vi "Global INIT.vi"() -> ()   [LabVIEW 2023]
uses:
  ctrl defs/ctrl arm motor.ctl
  ctrl defs/ctrl swerve motor.ctl
  ctrl defs/ctrl MOTOR SELECT.ctl
  <vilib>/Rock Robotics/WPI/ThirdParty/REV Robotics/REVLib/Typedef/Spark MAX Idle Mode.ctl
  ctrl defs/ctrl Spark MAX current limiting.ctl
  ctrl defs/ctrl motor PIDF coefficients.ctl
  <vilib>/Rock Robotics/WPI/ThirdParty/REV Robotics/REVLib/Typedef/Spark MAX Smart Motion Parameters.ctl
  ctrl defs/ctrl limit polarity.ctl
  <vilib>/Rock Robotics/WPI/ThirdParty/REV Robotics/REVLib/Typedef/Spark MAX Limit Switch Polarity.ctl
  ctrl defs/ctrl CANcoder.ctl
  ctrl defs/ctrl robot CG.ctl
  ctrl defs/ctrl XY coord.ctl
  ctrl defs/ctrl robot swerve dims.ctl
  ctrl defs/ctrl compressor begin.ctl
  ctrl defs/ctrl compressor config.ctl
  <vilib>/Rock Robotics/WPI/Compressor/WPI_CompressorFeedbackMode.ctl
  ctrl defs/ctrl solenoid.ctl
  <vilib>/Rock Robotics/WPI/Solenoid/WPI_SolenoidChannel.ctl
  <vilib>/Rock Robotics/WPI/Solenoid/WPI_SolenoidValue.ctl
  ctrl defs/ctrl DIO.ctl
  <vilib>/Rock Robotics/SystemInterfaces/DIO/FPGA_DIOChannel.ctl
  ctrl defs/ctrl LED init.ctl
  <vilib>/Rock Robotics/SystemInterfaces/DIO/FPGA_DIOPWMChannel.ctl
  ctrl defs/ctrl DEFINE GEAR.ctl
  ctrl defs/ctrl intake speeds.ctl
  ctrl defs/ctrl shooter speeds.ctl
panel:
  in  "Tab Control":T1(tab)=enum."ARMS"
  in  "DRIVE\nwheel diam (in)":dbl=4.0 format="%_4f"
  in  "swerve CANcoders":T2[](array[typedef])=[{"description"="front right", "Installed?"=TRUE, "CAN ID"=20, "CAN Bus"="rio", "refnum name"="FR ENC", "Sensor Direction"=FALSE, "Magnet Offset (Degrees)"=-264.1113, "gear ratio"=1.0}, {"description"="front left", "Installed?"=TRUE, "CAN ID"=21, "CAN Bus"="rio", "refnum name"="FL ENC", "Sensor Direction"=FALSE, "Magnet Offset (Degrees)"=-277.20703, "gear ratio"=1.0}, {"description"="rear left", "Installed?"=TRUE, "CAN ID"=22, "CAN Bus"="rio", "refnum name"="RL ENC", "Sensor Direction"=FALSE, "Magnet Offset (Degrees)"=-124.014, "gear ratio"=1.0}, {"description"="rear right", "Installed?"=TRUE, "CAN ID"=23, "CAN Bus"="rio", "refnum name"="RR ENC", "Sensor Direction"=FALSE, "Magnet Offset (Degrees)"=-162.158, "gear ratio"=1.0}] {"gear ratio" format="%_5f"}
  in  "swerve STEER motors":T3[](array[typedef])=[{"description"="front right", "MOTOR SELECT"=5676, "Installed?"=TRUE, "CAN ID"=3, "refnum name"="FR STEER", "Invert"=TRUE, "Idle Mode"=enum."Coast", "Current limiting"={"Linearized"=FALSE, "Free Speed (A)"=20.0, "Primay (A)"=40.0, "Limit RPM (0)"=0}, "MOTOR PIDF coefficients"={"PIDF"={"P Gain"=0.005, "I Gain"=0.0, "D Gain"=0.0, "F Gain"=0.0036, "I Zone"=0.0, "Min Output"=-1.0, "Max Output"=1.0}, "Smart Motion"={"Max Velocity"=1500.0, "Max Acceleration"=750.0, "Minimum Velocity Output"=0.1, "Allowed Closed Loop Error"=0.02}}, "gear ratio"=21.42857}, {"description"="front left", "MOTOR SELECT"=5676, "Installed?"=TRUE, "CAN ID"=9, "refnum name"="FL STEER", "Invert"=TRUE, "Idle Mode"=enum."Coast", "Current limiting"={"Linearized"=FALSE, "Free Speed (A)"=20.0, "Primay (A)"=40.0, "Limit RPM (0)"=0}, "MOTOR PIDF coefficients"={"PIDF"={"P Gain"=0.005, "I Gain"=0.0, "D Gain"=0.0, "F Gain"=0.0036, "I Zone"=0.0, "Min Output"=-1.0, "Max Output"=1.0}, "Smart Motion"={"Max Velocity"=1500.0, "Max Acceleration"=750.0, "Minimum Velocity Output"=0.1, "Allowed Closed Loop Error"=0.02}}, "gear ratio"=21.429}, {"description"="rear left", "MOTOR SELECT"=5676, "Installed?"=TRUE, "CAN ID"=8, "refnum name"="RL STEER", "Invert"=TRUE, "Idle Mode"=enum."Coast", "Current limiting"={"Linearized"=FALSE, "Free Speed (A)"=20.0, "Primay (A)"=40.0, "Limit RPM (0)"=0}, "MOTOR PIDF coefficients"={"PIDF"={"P Gain"=0.005, "I Gain"=0.0, "D Gain"=0.0, "F Gain"=0.0036, "I Zone"=0.0, "Min Output"=-1.0, "Max Output"=1.0}, "Smart Motion"={"Max Velocity"=1500.0, "Max Acceleration"=750.0, "Minimum Velocity Output"=0.1, "Allowed Closed Loop Error"=0.02}}, "gear ratio"=21.42857}, {"description"="rear right", "MOTOR SELECT"=5676, "Installed?"=TRUE, "CAN ID"=5, "refnum name"="RR STEER", "Invert"=TRUE, "Idle Mode"=enum."Coast", "Current limiting"={"Linearized"=FALSE, "Free Speed (A)"=20.0, "Primay (A)"=40.0, "Limit RPM (0)"=0}, "MOTOR PIDF coefficients"={"PIDF"={"P Gain"=0.005, "I Gain"=0.0, "D Gain"=0.0, "F Gain"=0.0036, "I Zone"=0.0, "Min Output"=-1.0, "Max Output"=1.0}, "Smart Motion"={"Max Velocity"=1500.0, "Max Acceleration"=750.0, "Minimum Velocity Output"=0.1, "Allowed Closed Loop Error"=0.02}}, "gear ratio"=21.42857}] {"gear ratio" format="%_5f"; "MOTOR SELECT" items=["REV NEO"=5676, "REV NEO 550"=11000, "VEX Falcon"=6380, "WC Kraken"=6000]}
  in  "swerve DRIVE motors":T3[](array[typedef])=[{"description"="front right", "MOTOR SELECT"=5676, "Installed?"=TRUE, "CAN ID"=4, "refnum name"="FR DRIVE", "Invert"=TRUE, "Idle Mode"=enum."Brake", "Current limiting"={"Linearized"=FALSE, "Free Speed (A)"=20.0, "Primay (A)"=40.0, "Limit RPM (0)"=0}, "MOTOR PIDF coefficients"={"PIDF"={"P Gain"=0.001, "I Gain"=0.0, "D Gain"=0.0, "F Gain"=0.0012, "I Zone"=0.0, "Min Output"=-1.0, "Max Output"=1.0}, "Smart Motion"={"Max Velocity"=1900.0, "Max Acceleration"=750.0, "Minimum Velocity Output"=0.1, "Allowed Closed Loop Error"=0.02}}, "gear ratio"=6.75}, {"description"="front left", "MOTOR SELECT"=5676, "Installed?"=TRUE, "CAN ID"=10, "refnum name"="FL DRIVE", "Invert"=TRUE, "Idle Mode"=enum."Brake", "Current limiting"={"Linearized"=FALSE, "Free Speed (A)"=20.0, "Primay (A)"=40.0, "Limit RPM (0)"=0}, "MOTOR PIDF coefficients"={"PIDF"={"P Gain"=0.001, "I Gain"=0.0, "D Gain"=0.0, "F Gain"=0.0012, "I Zone"=0.0, "Min Output"=-1.0, "Max Output"=1.0}, "Smart Motion"={"Max Velocity"=1900.0, "Max Acceleration"=750.0, "Minimum Velocity Output"=0.1, "Allowed Closed Loop Error"=0.02}}, "gear ratio"=6.75}, {"description"="rear left", "MOTOR SELECT"=5676, "Installed?"=TRUE, "CAN ID"=7, "refnum name"="RL DRIVE", "Invert"=TRUE, "Idle Mode"=enum."Brake", "Current limiting"={"Linearized"=FALSE, "Free Speed (A)"=20.0, "Primay (A)"=40.0, "Limit RPM (0)"=0}, "MOTOR PIDF coefficients"={"PIDF"={"P Gain"=0.001, "I Gain"=0.0, "D Gain"=0.0, "F Gain"=0.0012, "I Zone"=0.0, "Min Output"=-1.0, "Max Output"=1.0}, "Smart Motion"={"Max Velocity"=1900.0, "Max Acceleration"=750.0, "Minimum Velocity Output"=0.1, "Allowed Closed Loop Error"=0.02}}, "gear ratio"=6.75}, {"description"="rear right", "MOTOR SELECT"=5676, "Installed?"=TRUE, "CAN ID"=6, "refnum name"="RR DRIVE", "Invert"=TRUE, "Idle Mode"=enum."Brake", "Current limiting"={"Linearized"=FALSE, "Free Speed (A)"=20.0, "Primay (A)"=40.0, "Limit RPM (0)"=0}, "MOTOR PIDF coefficients"={"PIDF"={"P Gain"=0.001, "I Gain"=0.0, "D Gain"=0.0, "F Gain"=0.0012, "I Zone"=0.0, "Min Output"=-1.0, "Max Output"=1.0}, "Smart Motion"={"Max Velocity"=1900.0, "Max Acceleration"=750.0, "Minimum Velocity Output"=0.1, "Allowed Closed Loop Error"=0.02}}, "gear ratio"=6.75}] {"gear ratio" format="%_5f"; "MOTOR SELECT" items=["REV NEO"=5676, "REV NEO 550"=11000, "VEX Falcon"=6380, "WC Kraken"=6000]}
  in  "SOLENOIDS":T9[](array[typedef])=[{"description"="arm lock - BOTH", "Installed?"=TRUE, "refnum name"="LOCK - LEFT", "coils"=enum."Double", "forward channel"=enum."Solenoid 2", "reverse channel"=enum."Solenoid 3", "initial value"=enum."Reverse"}, {"description"="FLAP", "Installed?"=TRUE, "refnum name"="FLAP", "coils"=enum."Double", "forward channel"=enum."Solenoid 0", "reverse channel"=enum."Solenoid 1", "initial value"=enum."Reverse"}]
  in  "COMPRESSOR":T12={"description"="compressor", "Installed?"=TRUE, "refnum name"="COMP", "Feedback Configuration"={"Feedback Sensor"=enum."Digital Only", "Max Pressure (PSI)"=0.0, "Min Pressure (PSI)"=0.0}}
  in  "INTAKE speeds":T15={"forward"=1.0, "reverse"=-1.0} {"reverse" min=-1.0 max=-0.02 format="%.3f"; "forward" min=0.02 max=1.0 format="%.3f"}
  in  "INTAKE motor":T3={"description"="INTAKE", "MOTOR SELECT"=5676, "Installed?"=TRUE, "CAN ID"=11, "refnum name"="ref INTAKE", "Invert"=FALSE, "Idle Mode"=enum."Coast", "Current limiting"={"Linearized"=FALSE, "Free Speed (A)"=20.0, "Primay (A)"=40.0, "Limit RPM (0)"=0}, "MOTOR PIDF coefficients"={"PIDF"={"P Gain"=0.001, "I Gain"=0.0, "D Gain"=0.0, "F Gain"=0.0012, "I Zone"=0.0, "Min Output"=-1.0, "Max Output"=1.0}, "Smart Motion"={"Max Velocity"=1900.0, "Max Acceleration"=750.0, "Minimum Velocity Output"=0.1, "Allowed Closed Loop Error"=0.02}}, "gear ratio"=4.0} {"gear ratio" format="%_5f"; "MOTOR SELECT" items=["REV NEO"=5676, "REV NEO 550"=11000, "VEX Falcon"=6380, "WC Kraken"=6000]}
  in  "INTAKE GEAR TRAIN":T16[](array[typedef])=[{"DP"=20.0, "TEETH"=48, "DIAM (in)"=2.4, "rev"=FALSE, "ratio"=1.0}, {"DP"=20.0, "TEETH"=48, "DIAM (in)"=2.4, "rev"=TRUE, "ratio"=-1.0}, {"DP"=20.0, "TEETH"=20, "DIAM (in)"=1.0, "rev"=FALSE, "ratio"=0.4166666666666667}, {"DP"=20.0, "TEETH"=32, "DIAM (in)"=1.6, "rev"=TRUE, "ratio"=-0.6666666666666666}, {"DP"=20.0, "TEETH"=48, "DIAM (in)"=2.4, "rev"=FALSE, "ratio"=1.0}]
  in  "INTAKE ratio TO SMALL WHEEL":dbl=4.0
  in  "INTAKE ratio TO LARGE WHEEL":dbl=4.0
  in  "INTAKE wheel diam (in) - SM":dbl=2.25
  in  "INTAKE wheel diam (in) - LG":dbl=4.0
  out "K INTAKE":dbl=1.0 format="%#_13g"
  out "K LOADER":dbl=0.7272727272727272 format="%#_13g"
  in  "SHOOTER speeds":T17={"SPEAKER"=1.0, "AMP"=0.5} {"AMP" min=0.02 max=1.0 format="%.3f"; "SPEAKER" min=0.02 max=1.0 format="%.3f"}
  in  "DISABLE SHOOTER MECH":bool
  in  "SHOOTING motors":T3[](array[typedef])=[{"description"="SHOOTER CW MOTOR", "MOTOR SELECT"=11000, "Installed?"=TRUE, "CAN ID"=13, "refnum name"="ref SHOOTER", "Invert"=TRUE, "Idle Mode"=enum."Brake", "Current limiting"={"Linearized"=FALSE, "Free Speed (A)"=20.0, "Primay (A)"=40.0, "Limit RPM (0)"=0}, "MOTOR PIDF coefficients"={"PIDF"={"P Gain"=0.001, "I Gain"=0.0, "D Gain"=0.0, "F Gain"=0.0012, "I Zone"=0.0, "Min Output"=-1.0, "Max Output"=1.0}, "Smart Motion"={"Max Velocity"=1900.0, "Max Acceleration"=750.0, "Minimum Velocity Output"=0.1, "Allowed Closed Loop Error"=0.02}}, "gear ratio"=4.0}, {"description"="SHOOTER CCW follow", "MOTOR SELECT"=11000, "Installed?"=TRUE, "CAN ID"=14, "refnum name"="ref SHOOTER follow", "Invert"=TRUE, "Idle Mode"=enum."Brake", "Current limiting"={"Linearized"=FALSE, "Free Speed (A)"=20.0, "Primay (A)"=40.0, "Limit RPM (0)"=0}, "MOTOR PIDF coefficients"={"PIDF"={"P Gain"=0.001, "I Gain"=0.0, "D Gain"=0.0, "F Gain"=0.0012, "I Zone"=0.0, "Min Output"=-1.0, "Max Output"=1.0}, "Smart Motion"={"Max Velocity"=1900.0, "Max Acceleration"=750.0, "Minimum Velocity Output"=0.1, "Allowed Closed Loop Error"=0.02}}, "gear ratio"=4.0}] {"gear ratio" format="%_5f"; "MOTOR SELECT" items=["REV NEO"=5676, "REV NEO 550"=11000, "VEX Falcon"=6380, "WC Kraken"=6000]}
  in  "SHOOTER wheel diam (in)":dbl=4.0
  in  "ARM speeds":T15={"forward"=0.75, "reverse"=-0.75} {"reverse" min=-1.0 max=-0.02 format="%.3f"; "forward" min=0.02 max=1.0 format="%.3f"}
  in  "ARM motors":T18[](array[typedef])=[{" motor"={"description"="ARM-LEFT", "MOTOR SELECT"=5676, "Installed?"=TRUE, "CAN ID"=17, "refnum name"="ref ARM L", "Invert"=TRUE, "Idle Mode"=enum."Brake", "Current limiting"={"Linearized"=FALSE, "Free Speed (A)"=20.0, "Primay (A)"=40.0, "Limit RPM (0)"=0}, "MOTOR PIDF coefficients"={"PIDF"={"P Gain"=0.001, "I Gain"=0.0, "D Gain"=0.0, "F Gain"=0.0012, "I Zone"=0.0, "Min Output"=-1.0, "Max Output"=1.0}, "Smart Motion"={"Max Velocity"=1900.0, "Max Acceleration"=750.0, "Minimum Velocity Output"=0.1, "Allowed Closed Loop Error"=0.02}}, "gear ratio"=16.0}, "limit polarities"={"Forward limit"=enum."Normally Closed", "Reverse limit"=enum."Normally Closed"}, "MOTOR PIDF coefficients"={"PIDF"={"P Gain"=0.001, "I Gain"=0.0, "D Gain"=0.0, "F Gain"=0.0012, "I Zone"=0.0, "Min Output"=-1.0, "Max Output"=1.0}, "Smart Motion"={"Max Velocity"=1900.0, "Max Acceleration"=750.0, "Minimum Velocity Output"=0.1, "Allowed Closed Loop Error"=0.02}}}, {" motor"={"description"="ARM-RIGHT", "MOTOR SELECT"=5676, "Installed?"=TRUE, "CAN ID"=16, "refnum name"="ref ARM R", "Invert"=FALSE, "Idle Mode"=enum."Brake", "Current limiting"={"Linearized"=FALSE, "Free Speed (A)"=20.0, "Primay (A)"=40.0, "Limit RPM (0)"=0}, "MOTOR PIDF coefficients"={"PIDF"={"P Gain"=0.001, "I Gain"=0.0, "D Gain"=0.0, "F Gain"=0.0012, "I Zone"=0.0, "Min Output"=-1.0, "Max Output"=1.0}, "Smart Motion"={"Max Velocity"=1900.0, "Max Acceleration"=750.0, "Minimum Velocity Output"=0.1, "Allowed Closed Loop Error"=0.02}}, "gear ratio"=16.0}, "limit polarities"={"Forward limit"=enum."Normally Closed", "Reverse limit"=enum."Normally Closed"}, "MOTOR PIDF coefficients"={"PIDF"={"P Gain"=0.001, "I Gain"=0.0, "D Gain"=0.0, "F Gain"=0.0012, "I Zone"=0.0, "Min Output"=-1.0, "Max Output"=1.0}, "Smart Motion"={"Max Velocity"=1900.0, "Max Acceleration"=750.0, "Minimum Velocity Output"=0.1, "Allowed Closed Loop Error"=0.02}}}] {"motor"."gear ratio" format="%_5f"; "motor"."MOTOR SELECT" items=["REV NEO"=5676, "REV NEO 550"=11000, "VEX Falcon"=6380, "WC Kraken"=6000]}
  in  "LOADER max/min":T15={"forward"=1.0, "reverse"=-1.0} {"reverse" min=-1.0 max=-0.02 format="%.3f"; "forward" min=0.02 max=1.0 format="%.3f"}
  in  "LOADER speeds":T15={"forward"=0.64, "reverse"=-1.0} {"reverse" min=-1.0 max=-0.02 format="%.3f"; "forward" min=0.02 max=1.0 format="%.3f"}
  in  "LOADER wheel diam (in)":dbl=2.75
  in  "LOADING motors":T3[](array[typedef])=[{"description"="LOADING CW MOTOR", "MOTOR SELECT"=5676, "Installed?"=TRUE, "CAN ID"=12, "refnum name"="ref LOADER", "Invert"=FALSE, "Idle Mode"=enum."Brake", "Current limiting"={"Linearized"=FALSE, "Free Speed (A)"=20.0, "Primay (A)"=40.0, "Limit RPM (0)"=0}, "MOTOR PIDF coefficients"={"PIDF"={"P Gain"=0.001, "I Gain"=0.0, "D Gain"=0.0, "F Gain"=0.0012, "I Zone"=0.0, "Min Output"=-1.0, "Max Output"=1.0}, "Smart Motion"={"Max Velocity"=1900.0, "Max Acceleration"=750.0, "Minimum Velocity Output"=0.1, "Allowed Closed Loop Error"=0.02}}, "gear ratio"=4.0}, {"description"="LOADING CCW follow", "MOTOR SELECT"=5676, "Installed?"=TRUE, "CAN ID"=15, "refnum name"="ref LOADERS follow", "Invert"=TRUE, "Idle Mode"=enum."Brake", "Current limiting"={"Linearized"=FALSE, "Free Speed (A)"=20.0, "Primay (A)"=40.0, "Limit RPM (0)"=0}, "MOTOR PIDF coefficients"={"PIDF"={"P Gain"=0.001, "I Gain"=0.0, "D Gain"=0.0, "F Gain"=0.0012, "I Zone"=0.0, "Min Output"=-1.0, "Max Output"=1.0}, "Smart Motion"={"Max Velocity"=1900.0, "Max Acceleration"=750.0, "Minimum Velocity Output"=0.1, "Allowed Closed Loop Error"=0.02}}, "gear ratio"=4.0}] {"gear ratio" format="%_5f"; "MOTOR SELECT" items=["REV NEO"=5676, "REV NEO 550"=11000, "VEX Falcon"=6380, "WC Kraken"=6000]}
  in  "LED init":T21={"PWM Channel"=enum."PWM 0", "refnum name"="LED", "initial output"=0.51, "stack name"="LED/value", "Installed?"=FALSE}
  in  "DIO":T23[](array[typedef])=[{"description"="NOTE color sensor", "Installed?"=TRUE, "DIOChannel"=enum."DIO 0", "refnum name"="ref COLOR"}]
  in  "IMU OFFSET (deg)":dbl=90.0 format="%_4f"
  in  "swerve position coeff":T25(array[cluster])=[{"description"="front right", "wrt geom CTR"={"delX"=1, "delY"=1}}, {"description"="front left", "wrt geom CTR"={"delX"=-1, "delY"=1}}, {"description"="rear left", "wrt geom CTR"={"delX"=-1, "delY"=-1}}, {"description"="rear right", "wrt geom CTR"={"delX"=1, "delY"=-1}}]
  in  "ROBOT swerve dims":T26={"drive track"=24.428, "drive base"=24.428}
  in  "ROBOT CG":T27={"mass (lbm)"=103.39999999999999, "CG"={"X"=-0.11812379110251395, "Y"=-0.5906189555125736}, "Zcg"=24.0} {"CG"."Y" format="%.4g"; "CG"."X" format="%.4g"}
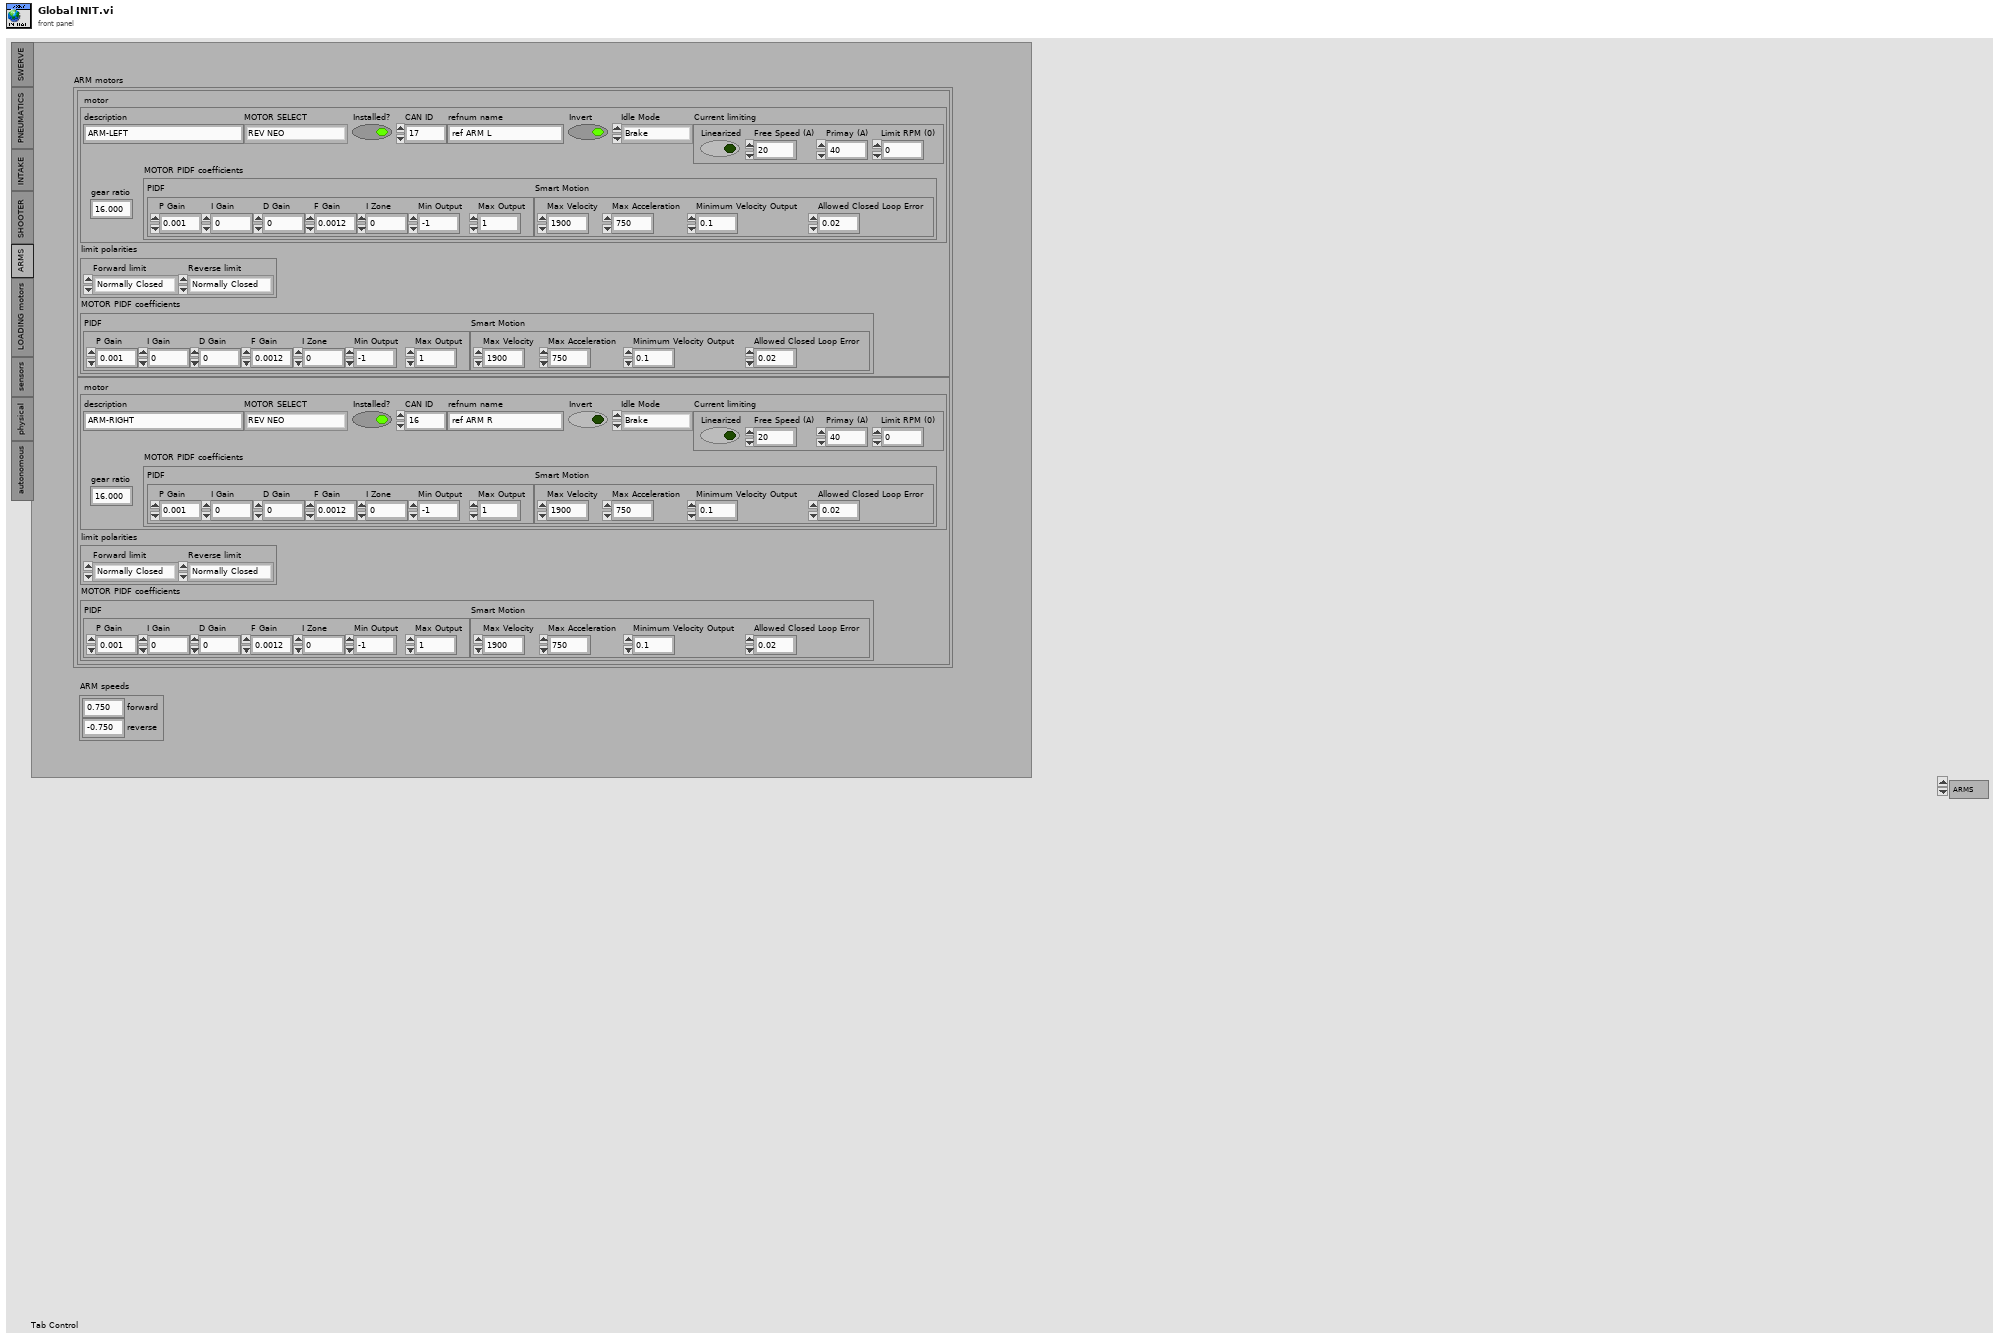
[diagram p1: front panel]
types:
  T1 = enum32{"SWERVE", "PNEUMATICS", "INTAKE ", "SHOOTER ", "ARMS", "LOADING motors", "sensors", "physical", "autonomous"}
  T2 = typedef "ctrl CANcoder.ctl" = cluster{"description":string, "Installed?":bool, "CAN ID":u8, "CAN Bus":string, "refnum name":string, "Sensor Direction":bool, "Magnet Offset (Degrees)":dbl, "gear ratio":dbl}
  T3 = typedef "ctrl swerve motor.ctl" = cluster{"description":string, "MOTOR SELECT":T4, "Installed?":bool, "CAN ID":u8, "refnum name":string, "Invert":bool, "Idle Mode":T5, "Current limiting":T6, "MOTOR PIDF coefficients":T7, "gear ratio":dbl}
  T4 = typedef "ctrl MOTOR SELECT.ctl" = i16
  T5 = typedef "Spark MAX Idle Mode.ctl" = enum16{"Coast", "Brake"}
  T6 = typedef "ctrl Spark MAX current limiting.ctl" = cluster{"Linearized":bool, "Free Speed (A)":dbl, "Primay (A)":dbl, "Limit RPM (0)":u32}
  T7 = typedef "ctrl motor PIDF coefficients.ctl" = cluster{"PIDF":cluster{"P Gain":dbl, "I Gain":dbl, "D Gain":dbl, "F Gain":dbl, "I Zone":dbl, "Min Output":dbl, "Max Output":dbl}, "Smart Motion":T8}
  T8 = typedef "Spark MAX Smart Motion Parameters.ctl" = cluster{"Max Velocity":dbl, "Max Acceleration":dbl, "Minimum Velocity Output":dbl, "Allowed Closed Loop Error":dbl}
  T9 = typedef "ctrl solenoid.ctl" = cluster{"description":string, "Installed?":bool, "refnum name":string, "coils":enum16{"Single", "Double"}, "forward channel":T10, "reverse channel":T10, "initial value":T11}
  T10 = typedef "WPI_SolenoidChannel.ctl" = enum8{"Solenoid 0", "Solenoid 1", "Solenoid 2", "Solenoid 3", "Solenoid 4", "Solenoid 5", "Solenoid 6", "Solenoid 7", "Solenoid 8", "Solenoid 9", "Solenoid 10", "Solenoid 11", "Solenoid 12", "Solenoid 13", "Solenoid 14", "Solenoid 15", "Invalid"}
  T11 = typedef "WPI_SolenoidValue.ctl" = enum16{"Off", "On", "Forward", "Reverse"}
  T12 = typedef "ctrl compressor begin.ctl" = cluster{"description":string, "Installed?":bool, "refnum name":string, "Feedback Configuration":T13}
  T13 = typedef "ctrl compressor config.ctl" = cluster{"Feedback Sensor":T14, "Max Pressure (PSI)":dbl, "Min Pressure (PSI)":dbl}
  T14 = typedef "WPI_CompressorFeedbackMode.ctl" = enum16{"Analog Only", "Digital Only", "Hybrid"}
  T15 = typedef "ctrl intake speeds.ctl" = cluster{"forward":dbl, "reverse":dbl}
  T16 = typedef "ctrl DEFINE GEAR.ctl" = cluster{"DP":dbl, "TEETH":i16, "DIAM (in)":dbl, "rev":bool, "ratio":dbl}
  T17 = typedef "ctrl shooter speeds.ctl" = cluster{"SPEAKER":dbl, "AMP":dbl}
  T18 = typedef "ctrl arm motor.ctl" = cluster{" motor":T3, "limit polarities":T19, "MOTOR PIDF coefficients":T7}
  T19 = typedef "ctrl limit polarity.ctl" = cluster{"Forward limit":T20, "Reverse limit":T20}
  T20 = typedef "Spark MAX Limit Switch Polarity.ctl" = enum16{"Normally Open", "Normally Closed"}
  T21 = typedef "ctrl LED init.ctl" = cluster{"PWM Channel":T22, "refnum name":string, "initial output":dbl, "stack name":string, "Installed?":bool}
  T22 = typedef "FPGA_DIOPWMChannel.ctl" = enum8{"PWM 0", "PWM 1", "PWM 2", "PWM 3", "PWM 4", "PWM 5", "PWM 6", "PWM 7", "PWM 8", "PWM 9", "PWM MXP 0", "PWM MXP 1", "PWM MXP 2", "PWM MXP 3", "PWM MXP 4", "PWM MXP 5", "PWM MXP 6", "PWM MXP 7", "PWM MXP 8", "PWM MXP 9", "Invalid"}
  T23 = typedef "ctrl DIO.ctl" = cluster{"description":string, "Installed?":bool, "DIOChannel":T24, "refnum name":string}
  T24 = typedef "FPGA_DIOChannel.ctl" = enum8{"DIO 0", "DIO 1", "DIO 2", "DIO 3", "DIO 4", "DIO 5", "DIO 6", "DIO 7", "DIO 8", "DIO 9", "DIO MXP 0", "DIO MXP 1", "DIO MXP 2", "DIO MXP 3", "DIO MXP 4", "DIO MXP 5", "DIO MXP 6", "DIO MXP 7", "DIO MXP 8", "DIO MXP 9", "DIO MXP 10", "DIO MXP 11", "DIO MXP 12", "DIO MXP 13", "DIO MXP 14", "DIO MXP 15", "SPI Port CS1", "SPI Port CS2", "SPI Port CS3", "SPI Port MISO", "SPI Port MOSI", "Invalid"}
  T25 = cluster{"description":string, "wrt geom CTR":cluster{"delX":i8, "delY":i8}}[]
  T26 = typedef "ctrl robot swerve dims.ctl" = cluster{"drive track":dbl, "drive base":dbl}
  T27 = typedef "ctrl robot CG.ctl" = cluster{"mass (lbm)":dbl, "CG":T28, "Zcg":dbl}
  T28 = typedef "ctrl XY coord.ctl" = cluster{"X":dbl, "Y":dbl}
diagram:
